vi "Configure Comparator.vi"(7 "Auxiliary Bin State (F:Disable)":bool, 8 "error in (no error)":errorcluster, 9 "Bin Count State (F:Disable)":bool, 10 "Comparator State (F:Disable)":bool, 11 "VISA resource name":refnum<visa-resource-name>) -> (0 "error out":errorcluster, 3 "VISA resource name out":refnum<visa-resource-name>)   [LabVIEW 2017, in "Agilent E4980.lvlib"]
doc: "Enables or disables the comparator, the auxiliary BIN, and the comparator BIN counting."
uses:
  Agilent E4980.lvlib
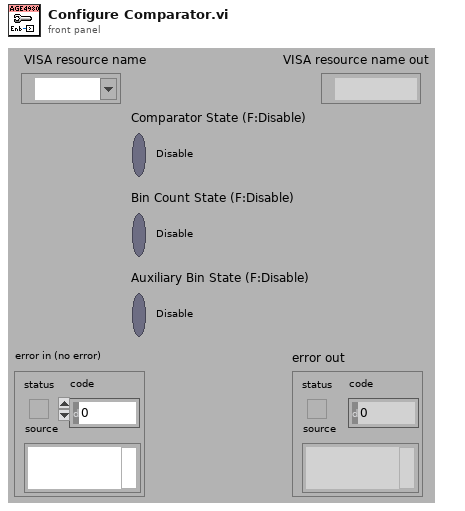
[diagram p1: front panel]
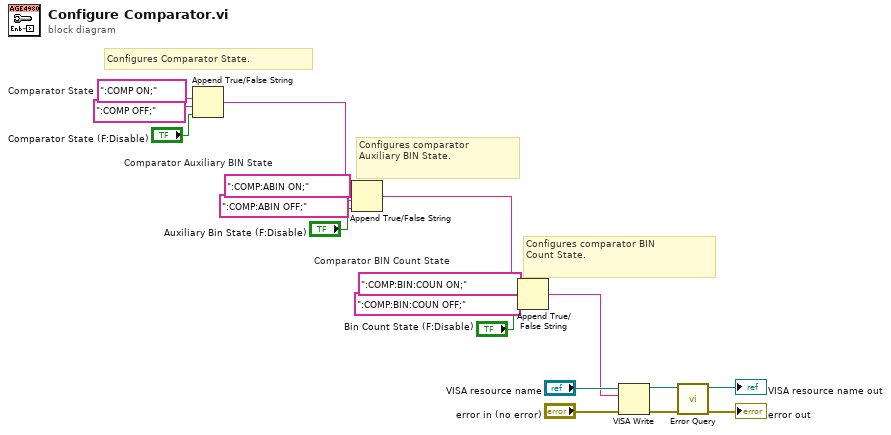
[diagram p0: block diagram]
diagram:
  w12 = ":COMP:BIN:COUN ON;"  # Comparator BIN Count State
  w15 = ":COMP:ABIN ON;"  # Comparator Auxiliary BIN State
  w17 = ":COMP ON;"  # Comparator State
  # "Configures comparator BIN\nCount State."
  # "Configures comparator\nAuxiliary BIN State."
  # "Configures Comparator State."
  n1 = Append True/False String(1:"Comparator State (F:Disable)", 2:":COMP OFF;" ("string (\"\")"), 3:w17) -> (0:w4:string)  [unwired: 1 in]
  n2 = Append True/False String(1:"Auxiliary Bin State (F:Disable)", 2:":COMP:ABIN OFF;" ("true string"), 3:w15, 4:w4) -> (0:w3:string)
  n3 = Append True/False String(1:"Bin Count State (F:Disable)", 2:":COMP:BIN:COUN OFF;" ("true string"), 3:w12, 4:w3) -> (0:w1:string)
  n4 = VISA Write(VISA resource name="VISA resource name", write buffer=w1, error in (no error)="error in (no error)") -> (VISA resource name out=w8:refnum<visa-resource-name>, error out=w7:errorcluster)  [unwired: 1 out]
  n5 = call "Error Query.vi"("error in (no error)"=w7, "VISA resource name"=w8) -> ("error out"=→"error out":errorcluster, "VISA resource name out"=→"VISA resource name out":refnum<visa-resource-name>)  [unwired: 6 in, 2 out]
